vi "beginStopPlayVSS.vi"(8 "error in (no error)":errorcluster, 10 "Game in":refnum<class "Game.lvclass">, 11 "StopPlayVSS in":refnum<class "StopPlayVSS.lvclass">) -> (0 "error out":errorcluster, 2 "Boolean":bool, 3 "StopPlayVSS out":refnum<class "StopPlayVSS.lvclass">)   [LabVIEW 2020, in "StopPlayVSS.lvclass"]
uses:
  StopPlayVSS.lvclass
  Game_class/Game.lvclass
  Command.ctl
  Game_class/Game.lvclass/Game.ctl
  Game_class/Read Referee.vi
  Referee_class/Referee.lvclass
panel:
  in  "queue":T1(array[ring])
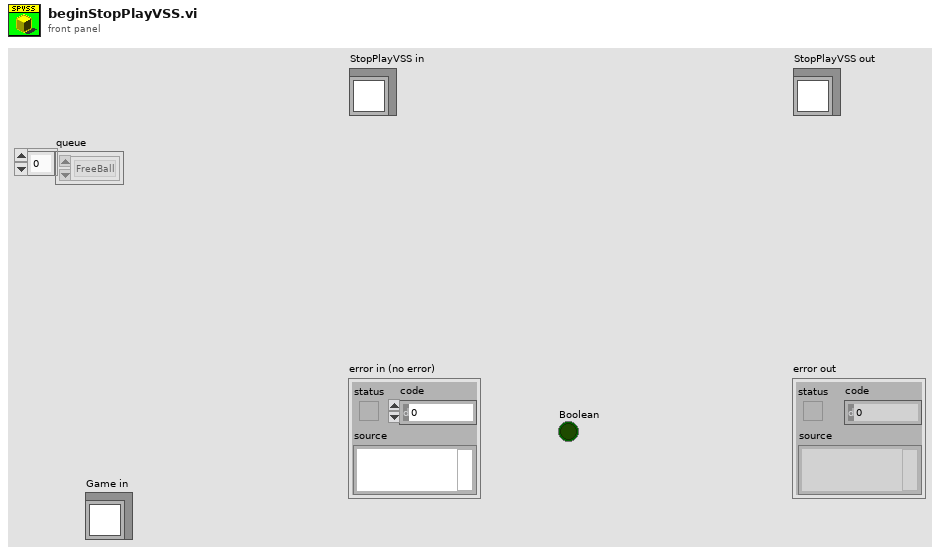
[diagram p1: front panel]
types:
  T1 = enum16{"FreeBall", "PrepareFreeBall", "GoalKickEnemy", "GoalKickAlly", "KickoffAlly", "KickoffEnemy", "PrepareGoalKickEnemy", "PrepareGoalKickAlly", "Stop", "PrepareKickoffEnemy", "PrepareKickoffAlly", "PreparePenaltyEnemy", "Timeout", "DeadBall", "NormalGame", "KickPenaltyAlly", "PenaltyEnemy", "BallChallenge", "PreparePenaltyAlly", "Halt"}[]
  T2 = typedef "Command.ctl" = enum16{"AUTO", "GAME_ON", "STOP", "HALT", "KICKOFF_ALLY", "KICKOFF_ENEMY", "FREE_BALL", "GOAL_KICK_ENEMY", "GOAL_KICK_ALLY", "PENALTY_KICK_ENEMY", "PENALTY_KICK_ALLY", "FREE_KICK"}
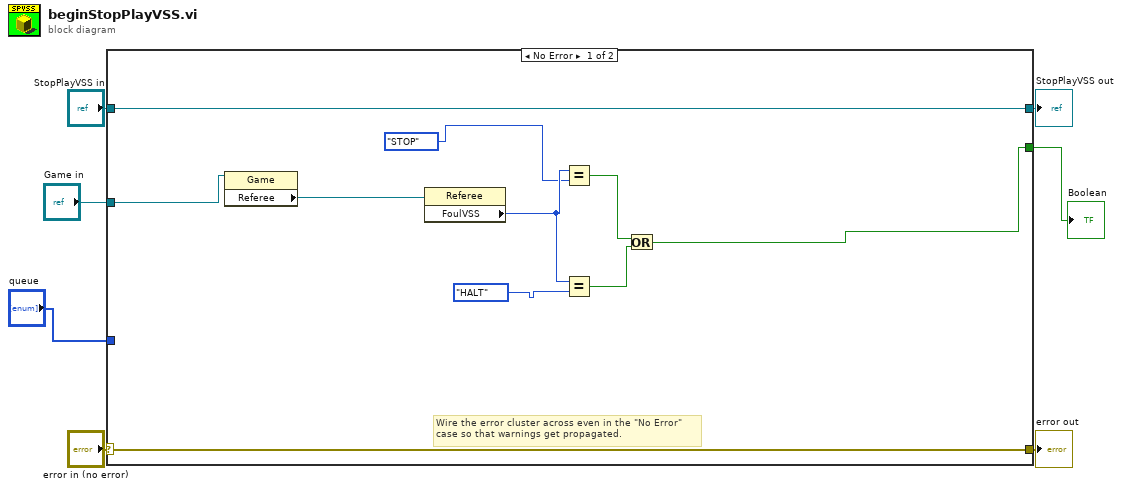
[diagram p0: block diagram]
diagram:
  n1 = case shown="No Error" "error in (no error)" {
    selector: "error in (no error)" -> [w16 w19]
    tunnel: [w16 w19] -> w6
    tunnel: [w17 w18] -> w4
    tunnel: "StopPlayVSS in" -> [w17 w18]
    tunnel: "Game in" -> [w14 _]
    tunnel: [w10 _] -> w2
    tunnel: "queue" -> [_ _]
    frame No Error {
      # "Wire the error cluster across even in the \"No Error\"\ncase so that warnings get propagated."
      n2 = property class="Game"(reference=w14) -> ("Referee"=w15:refnum<class "Referee.lvclass">)  [unwired: 1 in, 2 out]
      n3 = property class="Referee"(reference=w15) -> ("FoulVSS"=w13:T2)  [unwired: 1 in, 2 out]
      n4 = Equal?(x=w13, y=Command."STOP" ("FoulVSS")) -> (x = y?=w12:bool)
      n5 = Equal?(x=w13, y=Command."HALT" ("FoulVSS")) -> (x = y?=w11:bool)
      n6 = Or(x=w12, y=w11) -> (x .or. y?=w10:bool)
    }
    frame Error {
    }
  }
  "error out" <- w6
  "StopPlayVSS out" <- w4
  "Boolean" <- w2
